vi "zorder-not-respected.vi"() -> ()   [LabVIEW 2025]
panel:
  out "x+y":i32
  out "String out":string
  in  "y":i32
  in  "String in":string
  in  "Numeric":i32
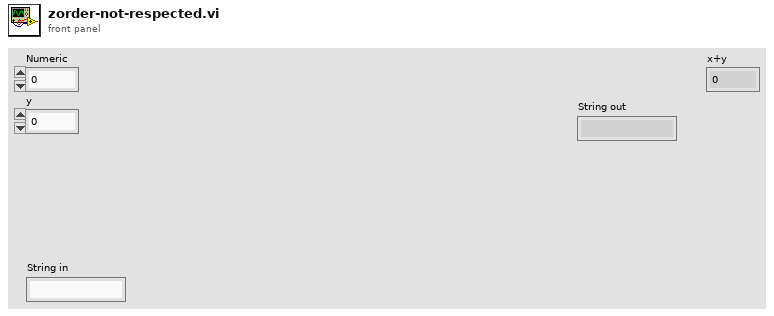
[diagram p1: front panel]
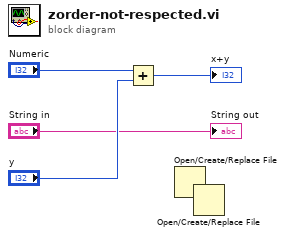
[diagram p0: block diagram]
diagram:
  n1 = Add(x="Numeric", y="y") -> (x+y=→"x+y":i32)
  n2 = Open/Create/Replace File() -> ()  [unwired: 6 in, 3 out]
  n3 = Open/Create/Replace File() -> ()  [unwired: 6 in, 3 out]
  "String out" <- "String in"
